vi "Begin.vi"(8 "error in":errorcluster) -> (0 "error out":errorcluster)   [LabVIEW 2017]
doc: "Called before other user functions, this VI is expected to open initial I/O refnums, load in file data, and do all program initialization. Notice that the <B>error out</B> terminal is simply used for data flow. Wiring it to other structures or subVIs ensures that this VI runs first."
uses:
  <vilib>/Rock Robotics/WPI/DriverStation/WPI_DriverStationRobotMode2.ctl
  <vilib>/Rock Robotics/WPI/SafetyOutput/WPI_SafetyOutputConfigMenu.ctl
  <vilib>/Rock Robotics/WPI/Solenoid/WPI_SolenoidChannel.ctl
  <vilib>/Rock Robotics/SystemInterfaces/DIO/FPGA_DIOChannel.ctl
  <vilib>/Rock Robotics/WPI/Encoder/WPI_EncoderType.ctl
  <vilib>/Rock Robotics/WPI/Joystick/WPI_JoystickDeviceEnum.ctl
  <vilib>/Rock Robotics/SystemInterfaces/DIO/FPGA_DIOPWMChannel.ctl
  Robot Global Data.vi
  <vilib>/Rock Robotics/Network Tables/NT Write String Array.vi
  <vilib>/Rock Robotics/WPI/RobotDrive/WPI_RobotDriveOpen4MotorWithExistingMotors.vi
  <vilib>/Rock Robotics/WPI/RobotDrive/WPI_RobotDriveOpen2MotorWithExistingMotors.vi
  <vilib>/Rock Robotics/WPI/Solenoid/WPI_SolenoidOpenSingle.vi
  <vilib>/Rock Robotics/WPI/Counter/WPI_CounterDigitalInputToDigitalSource.vi
  <vilib>/Rock Robotics/WPI/MotorControl/WPI_MotorControlOpen VictorSP.vi
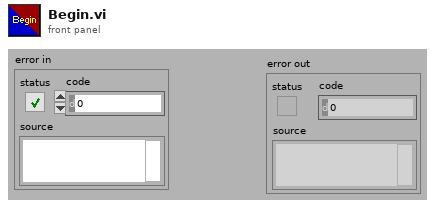
[diagram p1: front panel]
types:
  T1 = typedef "FPGA_DIOPWMChannel.ctl" = enum8{"PWM 0", "PWM 1", "PWM 2", "PWM 3", "PWM 4", "PWM 5", "PWM 6", "PWM 7", "PWM 8", "PWM 9", "PWM MXP 0", "PWM MXP 1", "PWM MXP 2", "PWM MXP 3", "PWM MXP 4", "PWM MXP 5", "PWM MXP 6", "PWM MXP 7", "PWM MXP 8", "PWM MXP 9", "Invalid"}
  T2 = typedef "WPI_JoystickDeviceEnum.ctl" = enum16{"USB 0", "USB 1", "USB 2", "USB 3", "USB 4", "USB 5"}
  T3 = typedef "WPI_EncoderType.ctl" = enum16{"1x", "2x", "4x"}
  T4 = typedef "FPGA_DIOChannel.ctl" = enum8{"DIO 0", "DIO 1", "DIO 2", "DIO 3", "DIO 4", "DIO 5", "DIO 6", "DIO 7", "DIO 8", "DIO 9", "DIO MXP 0", "DIO MXP 1", "DIO MXP 2", "DIO MXP 3", "DIO MXP 4", "DIO MXP 5", "DIO MXP 6", "DIO MXP 7", "DIO MXP 8", "DIO MXP 9", "DIO MXP 10", "DIO MXP 11", "DIO MXP 12", "DIO MXP 13", "DIO MXP 14", "DIO MXP 15", "SPI Port CS1", "SPI Port CS2", "SPI Port CS3", "SPI Port MISO", "SPI Port MOSI", "Invalid"}
  T5 = typedef "WPI_SolenoidChannel.ctl" = enum8{"Solenoid 0", "Solenoid 1", "Solenoid 2", "Solenoid 3", "Solenoid 4", "Solenoid 5", "Solenoid 6", "Solenoid 7", "Invalid"}
  T6 = typedef "WPI_SafetyOutputConfigMenu.ctl" = enum16{"Enable", "Disable"}
  T7 = typedef "WPI_DriverStationRobotMode2.ctl" = enum16{"Autonomous Disabled", "Autonomous Enabled", "Teleop Disabled", "Teleop Enabled", "Disconnected", "Finish", "Test Disabled", "Test Enabled", "Emergency Stopped"}
  T8 = typedef "WPI_MotorControlDeviceRef.ctl" = cluster{"DeviceStatus":errorcluster, "Type":T9, "PWM":cluster{"PWM Channel":T1, "DeadBand":T10}, "CAN":cluster{"Device Number":u8, "SetOutput VI Ref":variant, "GetOutput VI Ref":variant, "Enable VI Ref":variant, "Disable VI Ref":variant, "Data":variant}, "Invert":bool, "DIO PWM":cluster{"PWM \"Enable\" Channel":T1, "DIOChannel":T4, "PWM Rate":dbl}}
  T9 = typedef "WPI_MotorControlType.ctl" = enum16{"PWM", "CAN", "DIO PWM"}
  T10 = typedef "WPI_PWMDeadband.ctl" = cluster{"Name":string, "maxPositivePwm":i32, "minPositivePwm":i32, "centerPwm":i32, "maxNegativePwm":i32, "minNegativePwm":i32, "angularRange":u16}
  T11 = typedef "WPI_RobotDriveDevRef.ctl" = cluster{"DevStatus":errorcluster, "Motors[]":T8[], "Square Inputs":bool, "Max Output":dbl}
  T12 = typedef "WPI_SolenoidDevRef.ctl" = cluster{"DevStatus":errorcluster, "Pneumatics Control Module":u8, "Forward Solenoid Channel":T5, "Reverse Solenoid Channel":T5}
  T13 = typedef "WPI_DigitalInputDevRef.ctl" = cluster{"DevStatus":errorcluster, "DIO Channel":T4}
  T14 = typedef "FPGA_CounterEncoderSourceConvertionLVSourceType.ctl" = cluster{"DevStatus":errorcluster, "AnalogTriggerMode?":bool, "DigitalMode":cluster{"DIO Channel":T15}, "AnalogTriggerMode":cluster{"AnalogTriggerIndex":T16, "OutputType":T17}}
  T15 = typedef "FPGA_DIODigitalSourceChannel.ctl" = enum8{"DIO 0", "DIO 1", "DIO 2", "DIO 3", "DIO 4", "DIO 5", "DIO 6", "DIO 7", "DIO 8", "DIO 9", "DIO MXP 0", "DIO MXP 1", "DIO MXP 2", "DIO MXP 3", "DIO MXP 4", "DIO MXP 5", "DIO MXP 6", "DIO MXP 7", "DIO MXP 8", "DIO MXP 9", "DIO MXP 10", "DIO MXP 11", "DIO MXP 12", "DIO MXP 13", "DIO MXP 14", "DIO MXP 15", "Disabled"}
  T16 = typedef "FPGA_AnalogTriggerIndex.ctl" = enum8{"Trig 0", "Trig 1", "Trig 2", "Trig 3", "Trig 4", "Trig 5", "Trig 6", "Trig 7", "Invalid"}
  T17 = typedef "FPGA_AnalogTriggerOutType.ctl" = enum16{"InWindow", "TriggerState", "Rising", "Falling"}
  T18 = typedef "WPI_EncoderDevRef.ctl" = cluster{"DevStatus":errorcluster, "EncoderIndex":T19, "CounterIndex":T20, "DistancePerCount":dbl, "Decoding Type":T3}
  T19 = typedef "FPGA_EncoderIdx.ctl" = enum8{"Enc 0", "Enc 1", "Enc 2", "Enc 3", "Enc 4", "Enc 5", "Enc 6", "Enc 7", "Invalid"}
  T20 = typedef "FPGA_CounterCtrSystemIndex.ctl" = enum8{"Ctr 0", "Ctr 1", "Ctr 2", "Ctr 3", "Ctr 4", "Ctr 5", "Ctr 6", "Ctr 7", "Invalid"}
  T21 = typedef "WPI_JoystickDevRef.ctl" = cluster{"Device":T2}
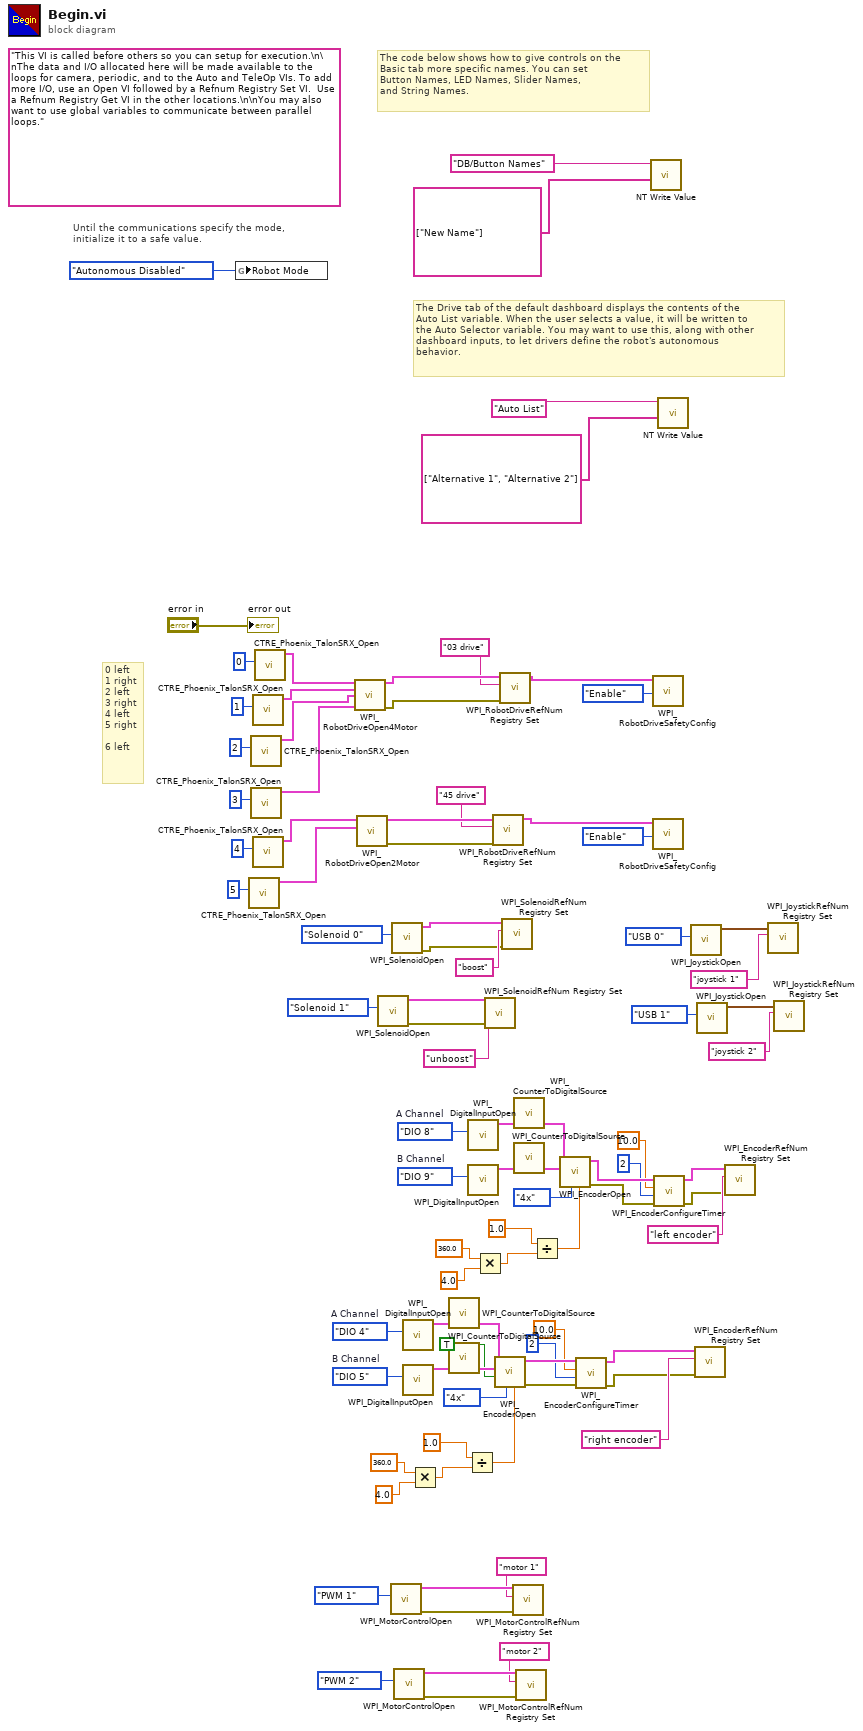
[diagram p0: block diagram]
diagram:
  w47 = FPGA_DIOChannel."DIO 5"  # B Channel
  w46 = FPGA_DIOChannel."DIO 4"  # A Channel
  w53 = FPGA_DIOChannel."DIO 9"  # B Channel
  w52 = FPGA_DIOChannel."DIO 8"  # A Channel
  (unwired) "This VI is called before others so you can setup for execution.\n\nThe data and I/O allocated here will be made available to the loops for camera, periodic, and to the Auto and TeleOp VIs. To add more I/O, use an Open VI followed by a Refnum Registry Set VI.  Use a Refnum Registry Get VI in the other locations.\n\nYou may also want to use global variables to communicate between parallel loops."
  # "0 left\n1 right\n2 left\n3 right\n4 left\n5 right \n\n6 left"
  # "The Drive tab of the default dashboard displays the contents of the\nAuto List variable. When the user selects a value, it will be written to\nthe Auto Selector variable. You may want to use this, along with other\ndashboard inputs, to let drivers define the robot's autonomous\nbehavior."
  # "The code below shows how to give controls on the\nBasic tab more specific names. You can set\nButton Names, LED Names, Slider Names,\nand String Names."
  # "Until the communications specify the mode,\ninitialize it to a safe value."
  n1 = global write "Robot Global Data.vi" "Robot Mode"(WPI_DriverStationRobotMode2."Autonomous Disabled" ("Robot Mode")) -> ()
  n2 = call <vilib>:"CTRE_Phoenix_TalonSRX_Open.vi"("Device Number"=u8 5) -> ("CAN Talon SRX Ref"=w72:T8)  [unwired: 9 in, 1 out]
  n3 = call <vilib>:"CTRE_Phoenix_TalonSRX_Open.vi"("Device Number"=u8 2) -> ("CAN Talon SRX Ref"=w75:T8)  [unwired: 9 in, 1 out]
  n4 = call <vilib>:"CTRE_Phoenix_TalonSRX_Open.vi"("Device Number"=u8 3) -> ("CAN Talon SRX Ref"=w74:T8)  [unwired: 9 in, 1 out]
  n5 = call <vilib>:"CTRE_Phoenix_TalonSRX_Open.vi"("Device Number"=u8 1) -> ("CAN Talon SRX Ref"=w76:T8)  [unwired: 9 in, 1 out]
  n6 = call <vilib>:"CTRE_Phoenix_TalonSRX_Open.vi"("Device Number"=u8 4) -> ("CAN Talon SRX Ref"=w73:T8)  [unwired: 9 in, 1 out]
  n7 = call <vilib>:"CTRE_Phoenix_TalonSRX_Open.vi"("Device Number"=u8 0) -> ("CAN Talon SRX Ref"=w77:T8)  [unwired: 9 in, 1 out]
  n8 = call-poly <vilib>:"WPI_RobotDriveOpen4Motor.vi"("Rear Left Motor Dev Ref"=w77, "Rear Right Motor Dev Ref"=w76, "Front Left Motor Dev Ref"=w75, "Front Right Motor Dev Ref"=w74) -> ("RobotDriveDevRef"=w71:T11, "error out"=w69:errorcluster)  [unwired: 10 in]
  n9 = call-poly <vilib>:"WPI_RobotDriveOpen2Motor.vi"("Right Motor Dev Ref"=w72, "Left Motor Dev Ref"=w73) -> ("error out"=w68:errorcluster, "RobotDriveDevRef"=w70:T11)  [unwired: 8 in]
  n10 = call-poly <vilib>:"WPI_SolenoidOpen.vi"("Solenoid Channel"=WPI_SolenoidChannel."Solenoid 1") -> ("error out"=w55:errorcluster, "SolenoidDevRef"=w59:T12)  [unwired: 9 in]
  n11 = call-poly <vilib>:"WPI_MotorControlOpen.vi"("PWM Channel"=FPGA_DIOPWMChannel."PWM 1") -> ("error out"=w12:errorcluster, "MotorControlDeviceRef"=w14:T8)  [unwired: 9 in]
  n12 = call-poly <vilib>:"WPI_SolenoidOpen.vi"("Solenoid Channel"=WPI_SolenoidChannel."Solenoid 0") -> ("error out"=w56:errorcluster, "SolenoidDevRef"=w58:T12)  [unwired: 9 in]
  n13 = call-poly <vilib>:"WPI_MotorControlOpen.vi"("PWM Channel"=FPGA_DIOPWMChannel."PWM 2") -> ("error out"=w16:errorcluster, "MotorControlDeviceRef"=w18:T8)  [unwired: 9 in]
  n14 = call <vilib>:"WPI_DigitalInputOpen.vi"("DIO Channel"=w46) -> ("DigitalInputDevRef"=w43:T13)  [unwired: 1 in, 9 out]
  n15 = call <vilib>:"WPI_DigitalInputOpen.vi"("DIO Channel"=w47) -> ("DigitalInputDevRef"=w44:T13)  [unwired: 1 in, 9 out]
  n16 = Multiply(x=360.0, y=4.0) -> (x*y=w2:dbl)
  n17 = call-poly <vilib>:"WPI_CounterToDigitalSource.vi"("DigitalInputDevRef"=w43) -> ("Digital Source"=w42:T14)  [unwired: 6 out]
  n18 = call-poly <vilib>:"WPI_CounterToDigitalSource.vi"("DigitalInputDevRef"=w44) -> ("Digital Source"=w45:T14)  [unwired: 6 out]
  n19 = Divide(x=1.0, y=w2) -> (x/y=w1:dbl)
  n20 = call <vilib>:"WPI_DigitalInputOpen.vi"("DIO Channel"=w52) -> ("DigitalInputDevRef"=w49:T13)  [unwired: 1 in, 9 out]
  n21 = call <vilib>:"WPI_DigitalInputOpen.vi"("DIO Channel"=w53) -> ("DigitalInputDevRef"=w50:T13)  [unwired: 1 in, 9 out]
  n22 = Multiply(x=360.0, y=4.0) -> (x*y=w7:dbl)
  n23 = call <vilib>:"WPI_SolenoidRefNum Registry Set.vi"("error in (no error)"=w55, "refnum name"="unboost", "SolenoidDevRef"=w59) -> ()  [unwired: 7 in, 2 out]
  n24 = call <vilib>:"WPI_RobotDriveRefNum Registry Set.vi"("error in (no error)"=w68, "refnum name"="45 drive", "RobotDriveDevRef"=w70) -> ("RobotDriveDevRef"=w64:T11)  [unwired: 7 in, 1 out]
  n25 = call <vilib>:"WPI_EncoderOpen.vi"("DistancePerCount"=w1, "Decoding Type"=WPI_EncoderType."4x", "Invert Direction (False)"=TRUE, "BSource"=w45, "ASource"=w42) -> ("error out"=w26:errorcluster, "EncoderDevRef"=w34:T18)  [unwired: 3 in, 2 out]
  n26 = call <vilib>:"WPI_RobotDriveRefNum Registry Set.vi"("error in (no error)"=w69, "refnum name"="03 drive", "RobotDriveDevRef"=w71) -> ("RobotDriveDevRef"=w66:T11)  [unwired: 7 in, 1 out]
  n27 = call <vilib>:"WPI_SolenoidRefNum Registry Set.vi"("error in (no error)"=w56, "refnum name"="boost", "SolenoidDevRef"=w58) -> ()  [unwired: 7 in, 2 out]
  n28 = call <vilib>:"WPI_MotorControlRefNum Registry Set.vi"("error in (no error)"=w12, "refnum name"="motor 1", "MotorControlDevRef"=w14) -> ()  [unwired: 7 in, 2 out]
  n29 = call-poly <vilib>:"WPI_CounterToDigitalSource.vi"("DigitalInputDevRef"=w49) -> ("Digital Source"=w48:T14)  [unwired: 6 out]
  n30 = call-poly <vilib>:"WPI_CounterToDigitalSource.vi"("DigitalInputDevRef"=w50) -> ("Digital Source"=w51:T14)  [unwired: 6 out]
  n31 = call <vilib>:"WPI_MotorControlRefNum Registry Set.vi"("error in (no error)"=w16, "refnum name"="motor 2", "MotorControlDevRef"=w18) -> ()  [unwired: 7 in, 2 out]
  n32 = Divide(x=1.0, y=w7) -> (x/y=w6:dbl)
  n33 = call <vilib>:"WPI_EncoderOpen.vi"("DistancePerCount"=w6, "Decoding Type"=WPI_EncoderType."4x", "BSource"=w51, "ASource"=w48) -> ("error out"=w38:errorcluster, "EncoderDevRef"=w37:T18)  [unwired: 4 in, 2 out]
  n34 = call <vilib>:"WPI_EncoderConfigureTimer.vi"("error in (no error)"=w26, "Number Samples to Average"=u8 2, "Minimum Rate"=10.0, "EncoderDevRef"=w34) -> ("error out"=w31:errorcluster, "EncoderDevRef"=w32:T18)  [unwired: 6 in]
  n35 = call-poly <vilib>:"NT Write Value.vi"("String Array"=string[] ["New Name"], "Name"="DB/Button Names") -> ()  [unwired: 9 in, 1 out]
  n36 = call <vilib>:"WPI_RobotDriveSafetyConfig.vi"("mode"=WPI_SafetyOutputConfigMenu."Enable", "RobotDriveDevRef"=w66) -> ()  [unwired: 8 in, 2 out]
  n37 = call <vilib>:"WPI_RobotDriveSafetyConfig.vi"("mode"=WPI_SafetyOutputConfigMenu."Enable", "RobotDriveDevRef"=w64) -> ()  [unwired: 8 in, 2 out]
  n38 = call <vilib>:"WPI_EncoderConfigureTimer.vi"("error in (no error)"=w38, "Number Samples to Average"=u8 2, "Minimum Rate"=10.0, "EncoderDevRef"=w37) -> ("error out"=w35:errorcluster, "EncoderDevRef"=w36:T18)  [unwired: 6 in]
  n39 = call-poly <vilib>:"NT Write Value.vi"("String Array"=string[] ["Alternative 1", "Alternative 2"], "Name"="Auto List") -> ()  [unwired: 9 in, 1 out]
  n40 = call <vilib>:"WPI_JoystickOpen.vi"("JoystickDevice"=WPI_JoystickDeviceEnum."USB 0") -> ("JoystickDevRef"=w25:T21)  [unwired: 10 in]
  n41 = call <vilib>:"WPI_EncoderRefNum Registry Set.vi"("error in (no error)"=w31, "refnum name"="right encoder", "EncoderDevRef"=w32) -> ()  [unwired: 7 in, 2 out]
  n42 = call <vilib>:"WPI_JoystickOpen.vi"("JoystickDevice"=WPI_JoystickDeviceEnum."USB 1") -> ("JoystickDevRef"=w22:T21)  [unwired: 10 in]
  n43 = call <vilib>:"WPI_EncoderRefNum Registry Set.vi"("error in (no error)"=w35, "refnum name"="left encoder", "EncoderDevRef"=w36) -> ()  [unwired: 7 in, 2 out]
  n44 = call <vilib>:"WPI_JoystickRefNum Registry Set.vi"("refnum name"="joystick 1", "JoystickDevRef"=w25) -> ()  [unwired: 8 in, 2 out]
  n45 = call <vilib>:"WPI_JoystickRefNum Registry Set.vi"("refnum name"="joystick 2", "JoystickDevRef"=w22) -> ()  [unwired: 8 in, 2 out]
  "error out" <- "error in"
